vi "Read Channels.vi"(8 "error in":errorcluster, 11 "cRIO repo in":refnum<class "_cRIORepo.lvclass">) -> (0 "error out":errorcluster, 2 "channels":T1[](array[typedef]), 3 "cRIO repo out":refnum<class "_cRIORepo.lvclass">)   [LabVIEW 2013, in "_cRIORepo.lvclass"]
uses:
  _cRIORepo.lvclass
  ChannelData.ctl
  _cRIORepo.lvclass/_cRIORepo.ctl
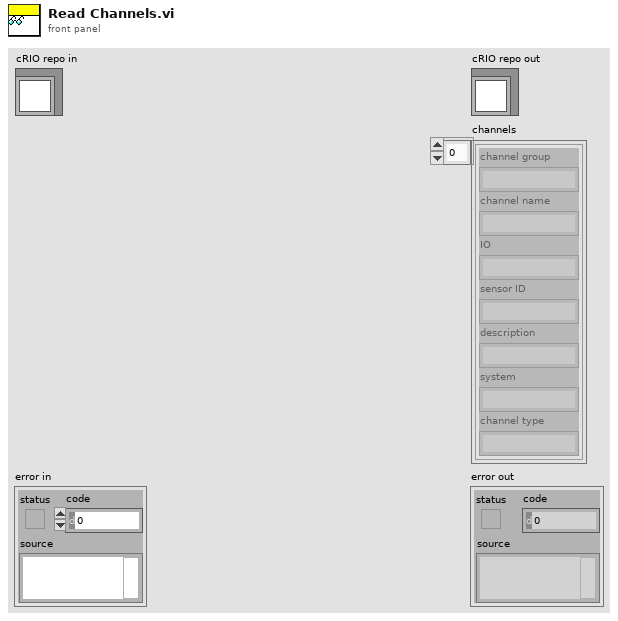
[diagram p1: front panel]
types:
  T1 = typedef "_cRIORepo.lvclass/ChannelData.ctl" = cluster{"channel group":string, "channel name":string, "IO ":string, "sensor ID":string, "description":string, "system":string, "channel type":string}
  T2 = typedef "cRIORepo.lvclass/ChannelData.ctl" = cluster{"channel group":string, "channel name":string, "IO ":string, "sensor ID":string, "description":string, "system":string, "channel type":string}
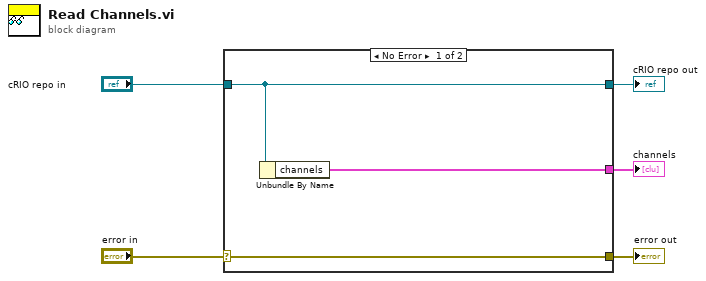
[diagram p0: block diagram]
diagram:
  n1 = case shown="No Error" "error in" {
    selector: "error in" -> [w8 w9]
    tunnel: [w8 w9] -> w4
    tunnel: [w7 w10] -> w2
    tunnel: "cRIO repo in" -> [w7 w10]
    tunnel: [w6 _] -> w1
    frame No Error {
      n2 = Unbundle By Name(w7) -> ("channels"=w6:T2[])
    }
    frame Error {
    }
  }
  "error out" <- w4
  "cRIO repo out" <- w2
  "channels" <- w1
